vi "CD Init_Prepare Inline Data_Complete Frame Descriptors.vi"(8 "error in (no error)":errorcluster, 10 "RTs In":T1[](array[typedef]) {"Mode Codes"."param item refs" format="%.0x"; "Mode Codes"."param block data refs"."Data Reference" format="%.0x"; "Mode Codes"."Timestamp Channel Data Reference" format="%.0x"; "subAddresses"."param item refs" format="%.0x"; "subAddresses"."param blocj data refs"."Data Reference" format="%.0x"; "subAddresses"."Timestamp Channel Data Reference" format="%.0x"; "Status Channel Data Reference" format="%.0x"; "Command Channels Refs" format="%.0x"}, 11 "Frames Descriptors In":T12[](array[typedef]) {"RT"."Status Channel Ref" format="%.0x"; "RT"."Words Block Data Refs"."Data Reference" format="%.0x"; "RT"."Timestamp Channel Data Reference" format="%.0x"; "BC"."Status Channel Refs" format="%.0x"; "BC"."param block data refs"."Data Reference" format="%.0x"; "BC"."Timestamp Channel Data Reference" format="%.0x"}) -> (0 "error out":errorcluster, 3 "Frames Descriptors Out":T12[](array[typedef]) {"RT"."Status Channel Ref" format="%.0x"; "RT"."Words Block Data Refs"."Data Reference" format="%.0x"; "RT"."Timestamp Channel Data Reference" format="%.0x"; "BC"."Status Channel Refs" format="%.0x"; "BC"."param block data refs"."Data Reference" format="%.0x"; "BC"."Timestamp Channel Data Reference" format="%.0x"})   [LabVIEW 2020, in "Ballard MIL-1553 Engine.lvlib"]
doc: "We complete Frame Descriptors for frames not defined in BC (or there is no BC)."
uses:
  Ballard MIL-1553 Engine.lvlib
  Controls/RT Inline Frame Descriptor.ctl
  Controls/RT Inline Frame Descriptor_BC.ctl
  <vilib>/NI VeriStand/Custom Device API/Data Reference.ctl
  <vilib>/NI VeriStand/Custom Device API/Block Data Reference.ctl
  <vilib>/NI VeriStand/Custom Device API/Custom Device Item Ref.ctl
  Shared/EncodeDecode/_typedefs/parameter_config_type.ctl
  Shared/EncodeDecode/_typedefs/parameter_config_type_type.ctl
  Shared/EncodeDecode/_typedefs/parameter_config_encoding_type.ctl
  Controls/RT Inline Frame Descriptor_RT.ctl
  Shared/Controls and Global/RT CWD2.ctl
  Shared/Controls and Global/RT CWD1.ctl
  Shared/Controls and Global/RT messageType.ctl
  Shared/Controls and Global/RT Remote Terminal.ctl
  Shared/Controls and Global/RT Remote Terminal_rtMode.ctl
  Shared/Controls and Global/RT Remote Terminal_RT subAddress.ctl
  Shared/Controls and Global/RT Remote Terminal_RT direction.ctl
  Shared/Controls and Global/RT Remote Terminal_RT Mode Code.ctl
  <vilib>/NI VeriStand/Custom Device Tools/Custom Device Utility Library/Custom Device Utility Library.lvlib
  Shared/Ballard 1553 Shared.lvlib
  <vilib>/NI VeriStand/Custom Device API/Custom Device API.lvlib
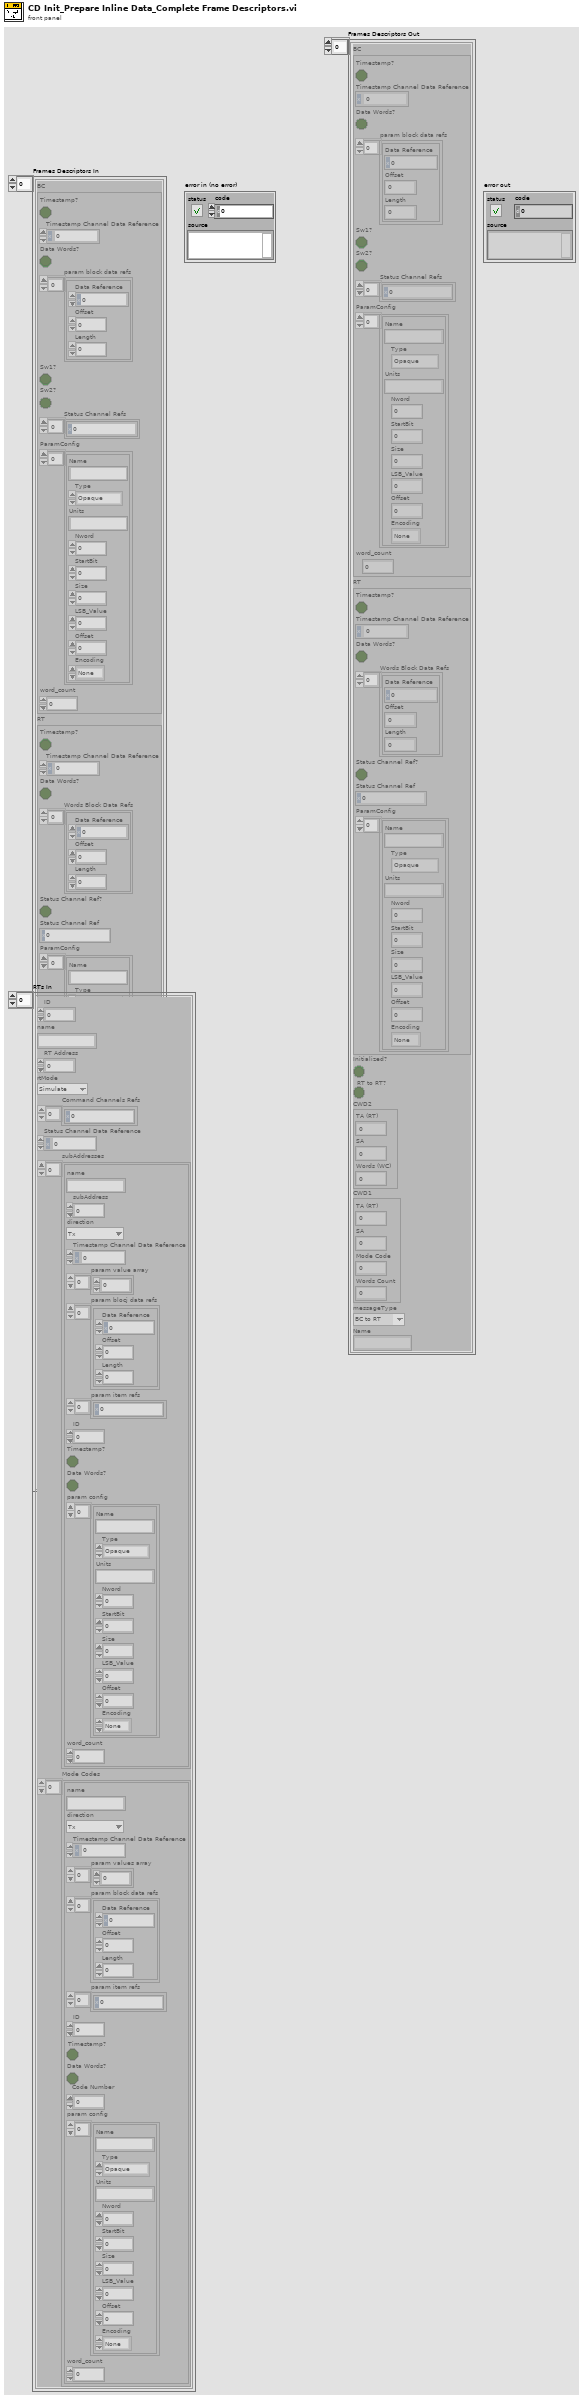
[diagram p1: front panel]
types:
  T1 = typedef "Ballard 1553 Shared.lvlib/RT Remote Terminal.ctl" = cluster{"ID":i32, "name":string, "RT Address":i32, "rtMode":T2, "Command Channels Refs":T3[], "Status Channel Data Reference":T4, "subAddresses":T5[], "Mode Codes":T11[]}
  T2 = typedef "Ballard 1553 Shared.lvlib/RT Remote Terminal_rtMode.ctl" = enum16{"Simulate", "Monitor", "Disable"}
  T3 = typedef "Custom Device API.lvlib/Custom Device Item Ref.ctl" = u64
  T4 = typedef "Custom Device API.lvlib/Data Reference.ctl" = i32
  T5 = typedef "Ballard 1553 Shared.lvlib/RT Remote Terminal_RT subAddress.ctl" = cluster{"name":string, "subAddress":i8, "direction":T6, "Timestamp Channel Data Reference":T4, "param value array":u16[], "param blocj data refs":T7[], "param item refs":T3[], "ID":i32, "Timestamp?":bool, "Data Words?":bool, "param config":T8[], "word_count":u8}
  T6 = typedef "Ballard 1553 Shared.lvlib/RT Remote Terminal_RT direction.ctl" = enum16{"Tx", "Rx"}
  T7 = typedef "Custom Device API.lvlib/Block Data Reference.ctl" = cluster{"Data Reference":T4, "Offset":u64, "Length":u64}
  T8 = typedef "parameter_config_type.ctl" = cluster{"Name":string, "Type":T9, "Units":string, "Nword":i32, "StartBit":i32, "Size":i32, "LSB_Value":i32, "Offset":i32, "Encoding":T10}
  T9 = typedef "parameter_config_type_type.ctl" = enum16{"Opaque", "Enum", "Float", "Integer", "Bcd", "Bool"}
  T10 = typedef "parameter_config_encoding_type.ctl" = enum16{"None", "2-complement", "Unsigned"}
  T11 = typedef "Ballard 1553 Shared.lvlib/RT Remote Terminal_RT Mode Code.ctl" = cluster{"name":string, "direction":T6, "Timestamp Channel Data Reference":T4, "param values array":u16[], "param block data refs":T7[], "param item refs":T3[], "ID":i32, "Timestamp?":bool, "Data Words?":bool, "Code Number":i32, "param config":T8[], "word_count":u8}
  T12 = typedef "Ballard MIL-1553 Engine.lvlib/RT Inline Frame Descriptor.ctl" = cluster{"BC":T13, "RT":T14, "Initialized?":bool, "RT to RT?":bool, "CWD2":T15, "CWD1":T16, "messageType":T17, "Name":string}
  T13 = typedef "Ballard MIL-1553 Engine.lvlib/RT Inline Frame Descriptor_BC.ctl" = cluster{"Timestamp?":bool, "Timestamp Channel Data Reference":T4, "Data Words?":bool, "param block data refs":T7[], "Sw1?":bool, "Sw2?":bool, "Status Channel Refs":T3[], "ParamConfig":T8[], "word_count":u8}
  T14 = typedef "Ballard MIL-1553 Engine.lvlib/RT Inline Frame Descriptor_RT.ctl" = cluster{"Timestamp?":bool, "Timestamp Channel Data Reference":T4, "Data Words?":bool, "Words Block Data Refs":T7[], "Status Channel Ref?":bool, "Status Channel Ref":T3, "ParamConfig":T8[]}
  T15 = typedef "Ballard 1553 Shared.lvlib/RT CWD2.ctl" = cluster{"TA (RT)":i8, "SA":i8, "Words (WC)":i8}
  T16 = typedef "Ballard 1553 Shared.lvlib/RT CWD1.ctl" = cluster{"TA (RT)":i8, "SA":i8, "Mode Code":i8, "Words Count":i8}
  T17 = typedef "Ballard 1553 Shared.lvlib/RT messageType.ctl" = enum16{"BC to RT", "RT to BC", "RT to RT", "MC (Rx)", "MC (Tx)"}
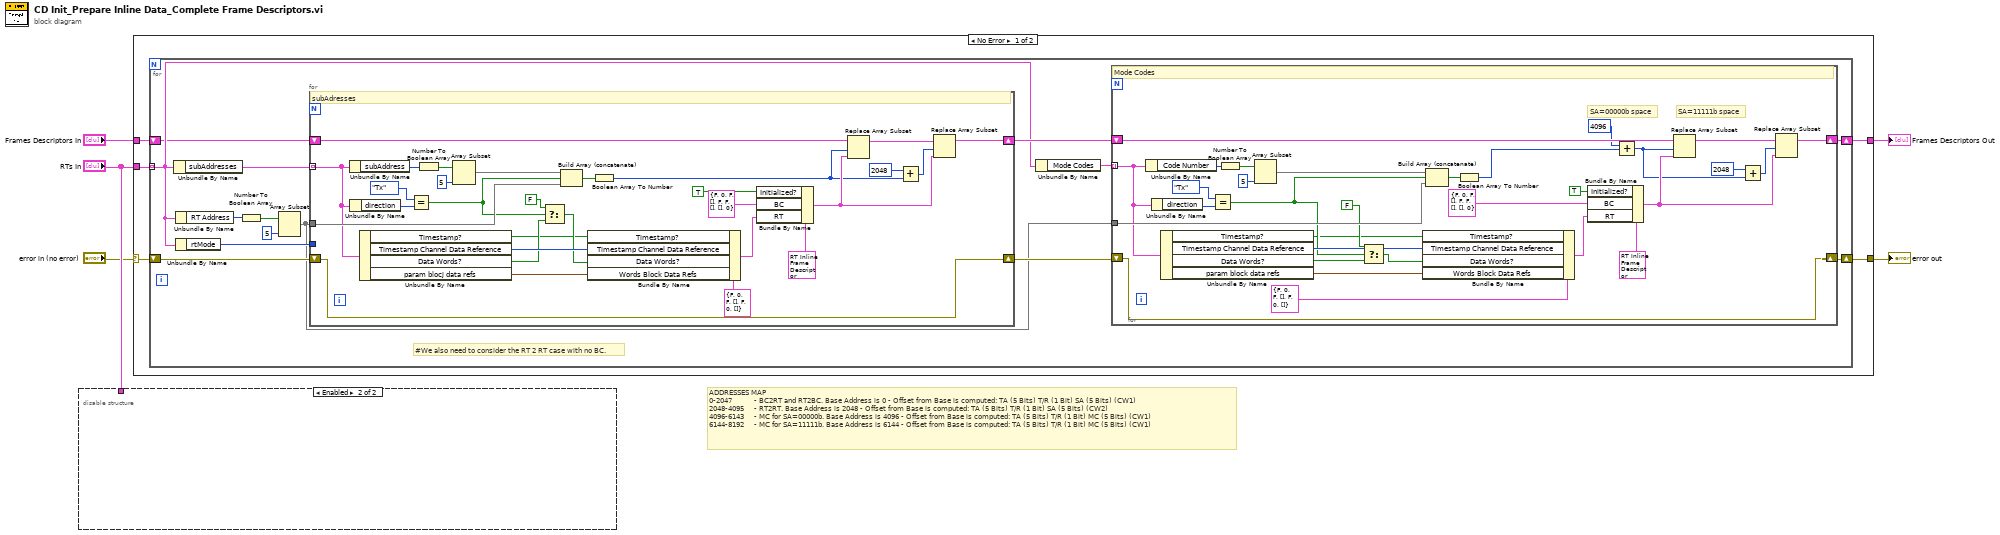
[diagram p0: block diagram]
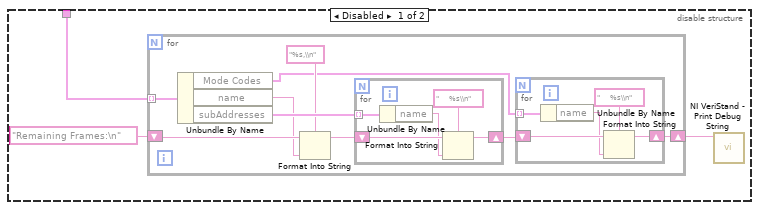
[diagram p2: hidden frame]
diagram:
  # "ADDRESSES MAP \n0-2047           - BC2RT and RT2BC. Base Address is 0 - Offset from Base is computed: TA (5 Bits) T/R (1 Bit) SA (5 Bits) (CW1)\n2048-4095     - RT2RT. Base Address is 2048 - Offset from Base is computed: TA (5 Bits) T/R (1 Bit) SA (5 Bits) (CW2)\n4096-6143     - MC for SA=00000b. Base Address is 4096 - Offset from Base is computed: TA (5 Bits) T/R (1 Bit) MC (5 Bits) (CW1)\n6144-8192     - MC for SA=11111b. Base Address is 6144 - Offset from Base is computed: TA (5 Bits) T/R (1 Bit) MC (5 Bits) (CW1)"
  n1 = disable-structure shown="Enabled" {
    disable-tunnel: "RTs In" -> [w8 _]
    frame Disabled {
      n2 = for {
        tunnel: w8 -> [w17] mode=indexing
        shift-right: [w11] -> w6
        shift-left: "Remaining Frames:\n" -> [w15]
        n3 = Unbundle By Name(w17) -> ("Mode Codes"=w9:T11[], "name"=w14:string, "subAddresses"=w16:T5[])
        n4 = Format Into String(format string="%s,\\n", initial string=w15, w14) -> (resulting string=w12:string)  [unwired: 1 in, 1 out]
        n5 = for {
          tunnel: w16 -> [w27] mode=indexing
          shift-right: [w26] -> w10
          shift-left: w12 -> [w25]
          n6 = Unbundle By Name(w27) -> ("name"=w24:string)
          n7 = Format Into String(format string="     %s\\n", initial string=w25, w24) -> (resulting string=w26:string)  [unwired: 1 in, 1 out]
        }
        n8 = for {
          tunnel: w9 -> [w22] mode=indexing
          shift-right: [w21] -> w11
          shift-left: w10 -> [w20]
          n9 = Unbundle By Name(w22) -> ("name"=w19:string)
          n10 = Format Into String(format string="     %s\\n", initial string=w20, w19) -> (resulting string=w21:string)  [unwired: 1 in, 1 out]
        }
      }
      n11 = call <vilib>:"NI VeriStand - Print Debug String.vi"("Message"=w6) -> ()  [unwired: 10 in, 1 out]
    }
    frame Enabled {
    }
  }
  n12 = case shown="No Error" "error in (no error)" {
    selector: "error in (no error)" -> [w28 w108]
    tunnel: [w32 w107] -> w5
    tunnel: "Frames Descriptors In" -> [w31 w107]
    tunnel: [w30 w108] -> w3
    tunnel: "RTs In" -> [w29 _]
    frame No Error {
      n13 = for {
        tunnel: w29 -> [w36] mode=indexing
        shift-right: [w39] -> w32
        shift-left: w31 -> [w33]
        shift-right: [w37] -> w30
        shift-left: w28 -> [w41]
        # "#We also need to consider the RT 2 RT case with no BC."
        n14 = Unbundle By Name(w36) -> ("subAddresses"=w43:T5[])
        n15 = Unbundle By Name(w36) -> ("RT Address"=w44:i32)
        n16 = Unbundle By Name(w36) -> ("rtMode"=w42:T2)
        n17 = Number To Boolean Array(number=w44) -> (Boolean array=w45:bool[])
        n18 = Array Subset(array=w45, length=5) -> (w34:bool[])  [unwired: 1 in]
        n19 = for {
          tunnel: w34 -> [w99]
          shift-right: [w90] -> w40
          shift-left: w33 -> [w87]
          tunnel: w43 -> [w94] mode=indexing
          tunnel: w42 -> [_]
          shift-right: [w88] -> w38
          shift-left: w41 -> [w88]
          # "subAdresses"
          n20 = Unbundle By Name(w94) -> ("subAddress"=w104:i8)
          n21 = Unbundle By Name(w94) -> ("direction"=w101:T6)
          n22 = Unbundle By Name(w94) -> ("Timestamp?"=w80:bool, "Timestamp Channel Data Reference"=w92:T4, "Data Words?"=w82:bool, "param blocj data refs"=w91:T7[])
          n23 = Equal?(x=RT_Remote_Terminal_RT_direction."Tx", y=w101) -> (x = y?=w84:bool)
          n24 = Number To Boolean Array(number=w104) -> (Boolean array=w105:bool[])
          n25 = Array Subset(array=w105, length=5) -> (w102:bool[])  [unwired: 1 in]
          n26 = Select(t=FALSE, s=w84, f=w82) -> (s? t:f=w81:bool)
          n27 = Build Array (concatenate)(w102, w84, w99) -> (w103:bool[])
          n28 = Bundle By Name(cluster=T14 {"Timestamp?"=FALSE, "Timestamp Channel Data Reference"=0, "Data Words?"=FALSE, "Words Block Data Refs"=[], "Status Channel Ref?"=FALSE, "Status Channel Ref"=0, "ParamConfig"=[]} ("RT"), "Timestamp?"=w80, "Timestamp Channel Data Reference"=w92, "Data Words?"=w81, "Words Block Data Refs"=w91) -> (w93:T14)
          n29 = Boolean Array To Number(Boolean array=w103) -> (number=w78:u16)
          n30 = Bundle By Name(cluster=T12 {"BC"={"Timestamp?"=FALSE, "Timestamp Channel Data Reference"=0, "Data Words?"=FALSE, "param block data refs"=[], "Sw1?"=FALSE, "Sw2?"=FALSE, "Status Channel Refs"=[], "ParamConfig"=[], "word_count"=0}, "RT"={"Timestamp?"=FALSE, "Timestamp Channel Data Reference"=0, "Data Words?"=FALSE, "Words Block Data Refs"=[], "Status Channel Ref?"=FALSE, "Status Channel Ref"=0, "ParamConfig"=[]}, "Initialized?"=FALSE, "RT to RT?"=FALSE, "CWD2"={"TA (RT)"=0, "SA"=0, "Words (WC)"=0}, "CWD1"={"TA (RT)"=0, "SA"=0, "Mode Code"=0, "Words Count"=0}, "messageType"=enum."BC to RT", "Name"=""} ("Frame Descriptor"), "Initialized?"=TRUE, "BC"=T13 {"Timestamp?"=FALSE, "Timestamp Channel Data Reference"=0, "Data Words?"=FALSE, "param block data refs"=[], "Sw1?"=FALSE, "Sw2?"=FALSE, "Status Channel Refs"=[], "ParamConfig"=[], "word_count"=0}, "RT"=w93) -> (w89:T12)
          n31 = Replace Array Subset(array=w87, new element=w89, index=w78) -> (w85:T12[])
          n32 = Add(x=u16 2048, y=w78) -> (x+y=w79:u16)
          n33 = Replace Array Subset(array=w85, new element=w89, index=w79) -> (w90:T12[])
        }
        n34 = Unbundle By Name(w36) -> ("Mode Codes"=w35:T11[])
        n35 = for {
          tunnel: w34 -> [w70]
          shift-right: [w60] -> w39
          shift-left: w40 -> [w69]
          tunnel: w35 -> [w64] mode=indexing
          shift-right: [w57] -> w37
          shift-left: w38 -> [w57]
          # "SA=11111b space"
          # "SA=00000b space"
          # "Mode Codes"
          n36 = Unbundle By Name(w64) -> ("Code Number"=w75:i32)
          n37 = Unbundle By Name(w64) -> ("direction"=w72:T6)
          n38 = Unbundle By Name(w64) -> ("Timestamp?"=w47:bool, "Timestamp Channel Data Reference"=w62:T4, "Data Words?"=w48:bool, "param block data refs"=w61:T7[])
          n39 = Equal?(x=RT_Remote_Terminal_RT_direction."Tx", y=w72) -> (x = y?=w51:bool)
          n40 = Number To Boolean Array(number=w75) -> (Boolean array=w76:bool[])
          n41 = Array Subset(array=w76, length=5) -> (w73:bool[])  [unwired: 1 in]
          n42 = Select(t=FALSE, s=w51, f=w48) -> (s? t:f=w49:bool)
          n43 = Bundle By Name(cluster=T14 {"Timestamp?"=FALSE, "Timestamp Channel Data Reference"=0, "Data Words?"=FALSE, "Words Block Data Refs"=[], "Status Channel Ref?"=FALSE, "Status Channel Ref"=0, "ParamConfig"=[]} ("RT"), "Timestamp?"=w47, "Timestamp Channel Data Reference"=w62, "Data Words?"=w49, "Words Block Data Refs"=w61) -> (w63:T14)
          n44 = Build Array (concatenate)(w73, w51, w70) -> (w74:bool[])
          n45 = Boolean Array To Number(Boolean array=w74) -> (number=w58:u16)
          n46 = Bundle By Name(cluster=T12 {"BC"={"Timestamp?"=FALSE, "Timestamp Channel Data Reference"=0, "Data Words?"=FALSE, "param block data refs"=[], "Sw1?"=FALSE, "Sw2?"=FALSE, "Status Channel Refs"=[], "ParamConfig"=[], "word_count"=0}, "RT"={"Timestamp?"=FALSE, "Timestamp Channel Data Reference"=0, "Data Words?"=FALSE, "Words Block Data Refs"=[], "Status Channel Ref?"=FALSE, "Status Channel Ref"=0, "ParamConfig"=[]}, "Initialized?"=FALSE, "RT to RT?"=FALSE, "CWD2"={"TA (RT)"=0, "SA"=0, "Words (WC)"=0}, "CWD1"={"TA (RT)"=0, "SA"=0, "Mode Code"=0, "Words Count"=0}, "messageType"=enum."BC to RT", "Name"=""} ("Frame Descriptor"), "Initialized?"=TRUE, "BC"=T13 {"Timestamp?"=FALSE, "Timestamp Channel Data Reference"=0, "Data Words?"=FALSE, "param block data refs"=[], "Sw1?"=FALSE, "Sw2?"=FALSE, "Status Channel Refs"=[], "ParamConfig"=[], "word_count"=0}, "RT"=w63) -> (w59:T12)
          n47 = Add(x=u16 4096, y=w58) -> (x+y=w55:u16)
          n48 = Replace Array Subset(array=w69, new element=w59, index=w55) -> (w56:T12[])
          n49 = Add(x=u16 2048, y=w55) -> (x+y=w53:u16)
          n50 = Replace Array Subset(array=w56, new element=w59, index=w53) -> (w60:T12[])
        }
      }
    }
    frame Error {
    }
  }
  "Frames Descriptors Out" <- w5
  "error out" <- w3
